vi "VerifLimitesConditionsFonctionnelles.vi"(8 "Limite inférieure":T1 {"Valeur" format="%f"}, 11 "Limite supérieure":T1 {"Valeur" format="%f"}) -> (2 "Limites OK ?":bool)   [LabVIEW 2013]
uses:
  LIBRAIRIE/010_DATABASE/50_STATISTIQUES/020_STATISTIQUES/Ctrl/STAT_Limite.ctl
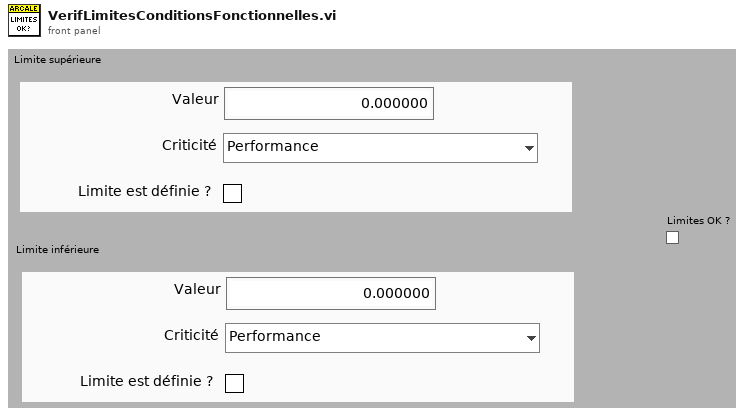
[diagram p1: front panel]
types:
  T1 = typedef "STAT_Limite.ctl" = cluster{"Valeur":dbl, "Criticité":T2, "Limite est définie ?":bool}
  T2 = typedef "STAT_Enum_Criticité.ctl" = enum16{"Performance", "Working", "Safety"}
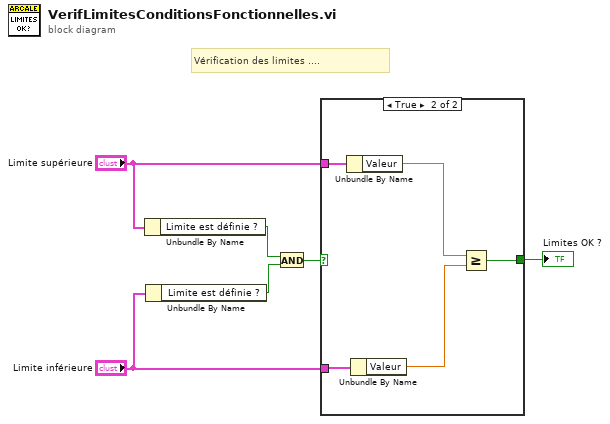
[diagram p0: block diagram]
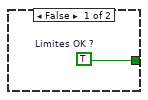
[diagram p2: hidden frame]
diagram:
  # "Vérification des limites ...."
  n1 = Unbundle By Name("Limite supérieure") -> ("Limite est définie ?"=w6:bool)
  n2 = Unbundle By Name("Limite inférieure") -> ("Limite est définie ?"=w5:bool)
  n3 = And(x=w6, y=w5) -> (x .and. y?=w4:bool)
  n4 = case shown="True" w4 {
    tunnel: "Limite supérieure" -> [_ w12]
    tunnel: "Limite inférieure" -> [_ w11]
    tunnel: [w7 w8] -> w1
    frame False {
      w7 = TRUE  # Limites OK ?
    }
    frame True {
      n5 = Unbundle By Name(w12) -> ("Valeur"=w10:dbl)
      n6 = Unbundle By Name(w11) -> ("Valeur"=w9:dbl)
      n7 = Greater Or Equal?(x=w10, y=w9) -> (x >= y?=w8:bool)
    }
  }
  "Limites OK ?" <- w1
